vi "VCO.vi"(8 "sampling frequency":dbl=0.1, 10 "center frequency":dbl[](array[numeric]), 11 "X":dbl[](array[numeric])) -> (0 "error":i32, 3 "Y":dbl[](array[numeric]))   [LabVIEW 2020, in "NI_AALBase.lvlib"]
uses:
  NI_AALBase.lvlib
panel:
  # "Voltage Controlled Oscillator"
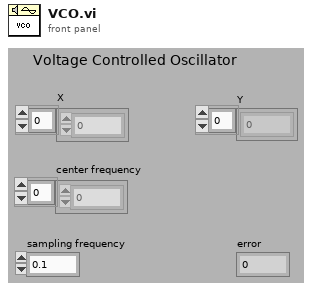
[diagram p1: front panel]
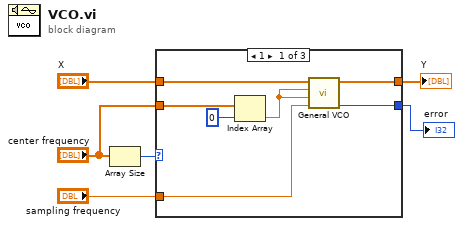
[diagram p0: block diagram]
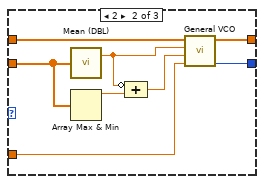
[diagram p2: hidden frame]
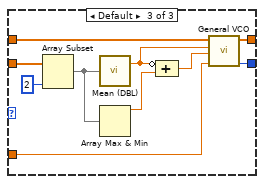
[diagram p3: hidden frame]
diagram:
  n1 = Array Size(array="center frequency") -> (size(s)=w1:i32)
  n2 = case shown="1" w1 {
    tunnel: "center frequency" -> [w13 w15 w26]
    tunnel: "X" -> [w11 w19 w31]
    tunnel: "sampling frequency" -> [w10 w17 w28]
    tunnel: [w9 w21 w30] -> w3
    tunnel: [w8 w20 w29] -> w2
    frame 1 {
      n3 = Index Array(array=w13, index=0) -> (element=w7:dbl)
      n4 = call "General VCO.vi"("fs"=w10, "range"=w7, "center frequency"=w7, "X"=w11) -> ("error"=w8:i32, "Y"=w9:dbl[])  [unwired: 6 in]
    }
    frame 2 {
      n5 = call "Mean (DBL).vi"("X"=w15) -> ("mean"=w18:dbl)  [unwired: 1 out]
      n6 = Array Max & Min(array=w15) -> (max value=w14:dbl)  [unwired: 3 out]
      n7 = Compound Arithmetic op=ADD(invert w18, w14) -> (w16:dbl)
      n8 = call "General VCO.vi"("fs"=w17, "range"=w16, "center frequency"=w18, "X"=w19) -> ("error"=w20:i32, "Y"=w21:dbl[])  [unwired: 6 in]
    }
    frame Default {
      n9 = Array Subset(array=w26, length=2) -> (w24:dbl[])  [unwired: 1 in]
      n10 = call "Mean (DBL).vi"("X"=w24) -> ("mean"=w25:dbl)  [unwired: 1 out]
      n11 = Array Max & Min(array=w24) -> (max value=w27:dbl)  [unwired: 3 out]
      n12 = Compound Arithmetic op=ADD(invert w25, w27) -> (w22:dbl)
      n13 = call "General VCO.vi"("fs"=w28, "range"=w22, "center frequency"=w25, "X"=w31) -> ("error"=w29:i32, "Y"=w30:dbl[])  [unwired: 6 in]
    }
  }
  "Y" <- w3
  "error" <- w2
